vi "Example String Functions 2.vi"(8 "Error In":errorcluster) -> (0 "Error Out":errorcluster)   [LabVIEW 2014]
panel:
  out "number 2":dbl
  out "F-format string":string
  out "number":i32
  out "offset past number":i32
  out "decimal integer string":string
  out "offset past match":i32
  out "after substring":string
  out "match substring":string
  out "before substring":string
  out "substring":string
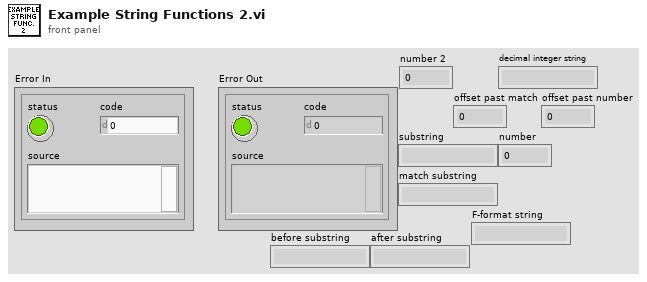
[diagram p1: front panel]
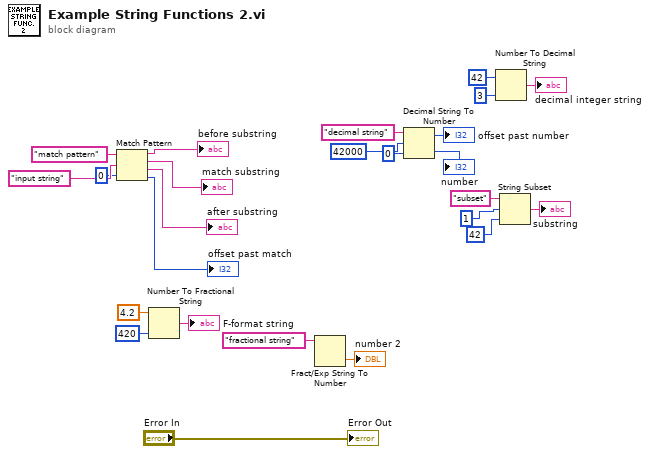
[diagram p0: block diagram]
diagram:
  n1 = Match Pattern(string="match pattern", regular expression="input string", offset (0)=0) -> (before substring=→"before substring":string, match substring=→"match substring":string, after substring=→"after substring":string, offset past match=→"offset past match":i32)
  n2 = Number To Fractional String(number=4.2, precision (6)=i16 420) -> (F-format string=→"F-format string":string)  [unwired: 2 in]
  n3 = Fract/Exp String To Number(string="fractional string") -> (number=→"number 2":dbl)  [unwired: 3 in, 1 out]
  n4 = Decimal String To Number(string="decimal string", offset=42000, default (0L)=0 ("default (0 I32)")) -> (offset past number=→"offset past number":i32, number=→"number":i32)
  n5 = Number To Decimal String(number=42, width (-)=i16 3) -> (decimal integer string=→"decimal integer string":string)
  n6 = String Subset(string="subset", offset (0)=1, length (rest)=42 ("length (rest)")) -> (substring=→"substring":string)
  "Error Out" <- "Error In"
